vi "CalculateSSDImages.vi"(10 "Template":T1, 11 "Image":T1) -> (3 "SSD":dbl[][](array[numeric]))   [LabVIEW 2014]
uses:
  <vilib>/vision/Image Controls.llb/IMAQ Image.ctl
  LocalQuadraticSumImages.vi
  FrequencyDomainCorrelationImages.vi
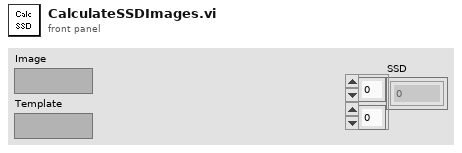
[diagram p1: front panel]
types:
  T1 = typedef "IMAQ Image.ctl" = refnum<image>
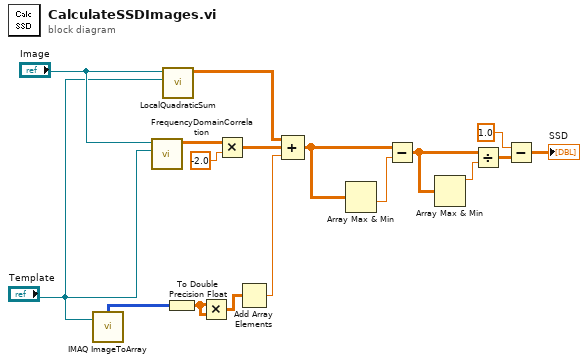
[diagram p0: block diagram]
diagram:
  n1 = call "IMAQ ImageToArray"("Image"="Template") -> ("Image Pixels (U8)"=w6:u8[][])  [unwired: 3 in, 4 out]
  n2 = call-poly "FrequencyDomainCorrelation.vi"("Template"="Template", "Image"="Image") -> ("FDCorrelation"=w7:sgl[][])  [unwired: 9 in]
  n3 = call-poly "LocalQuadraticSum.vi"("Template"="Template", "Image"="Image") -> ("localsum"=w1:dbl[][])  [unwired: 9 in]
  n4 = To Double Precision Float(number=w6) -> (double precision float=w5:dbl[][])
  n5 = Multiply(x=w5, y=w5) -> (x*y=w4:dbl[][])
  n6 = Multiply(x=w7, y=-2.0) -> (x*y=w15:dbl[][])
  n7 = Add Array Elements(numeric array=w4) -> (sum=w16:dbl)
  n8 = Compound Arithmetic op=ADD(w1, w15, w16) -> (w14:dbl[][])
  n9 = Array Max & Min(array=w14) -> (min value=w13:dbl)  [unwired: 3 out]
  n10 = Subtract(x=w14, y=w13) -> (x-y=w10:dbl[][])
  n11 = Array Max & Min(array=w10) -> (max value=w11:dbl)  [unwired: 3 out]
  n12 = Divide(x=w10, y=w11) -> (x/y=w9:dbl[][])
  n13 = Subtract(x=1.0, y=w9) -> (x-y=→"SSD":dbl[][])
